vi "Set Active Objective.vi"(8 "error in (no error)":errorcluster {"code" format="%.0x"}, 9 "Objective Number (1)":i32=1, 10 "Device Number (1)":i32=1, 11 "VISA Resource Name":refnum<visa-resource-name>) -> (0 "error out":errorcluster {"code" format="%.0x"}, 3 "VISA Resource Name Out":refnum<visa-resource-name>)   [LabVIEW 2018, in "Olympus IX BX Series.lvlib"]
doc: "Engages the objective sin the specified revolving nosepiece position into the light axis."
uses:
  Olympus IX BX Series.lvlib
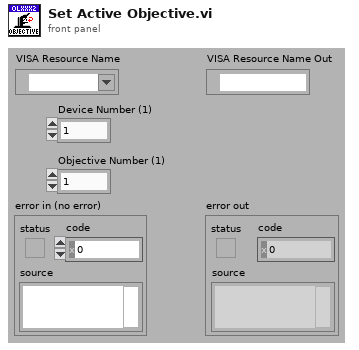
[diagram p1: front panel]
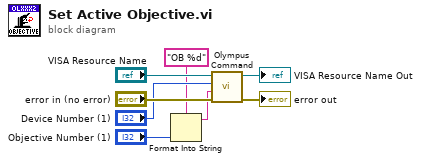
[diagram p0: block diagram]
diagram:
  n1 = Format Into String(format string="OB %d", "Objective Number (1)") -> (resulting string=w5:string)  [unwired: 2 in, 1 out]
  n2 = call "Olympus Command.vi"("error in (no error)"="error in (no error)", "Command string"=w5, "Device Number (1)"="Device Number (1)", "VISA Resource Name"="VISA Resource Name") -> ("error out"=→"error out":errorcluster, "VISA Resource Name Out"=→"VISA Resource Name Out":refnum<visa-resource-name>)  [unwired: 5 in, 1 out]
